vi "PCTrig.vi"(0 "object in":refnum<class "AD2_SDK.lvclass">, 5 "error in (no error)":errorcluster) -> (14 "object out":refnum<class "AD2_SDK.lvclass">, 19 "error out":errorcluster)   [LabVIEW 2019, in "AD2_SDK.lvclass"]
uses:
  AD2_SDK.lvclass
  Olasdwf/Olasdwf.lvlib
panel:
  out "function return":i32
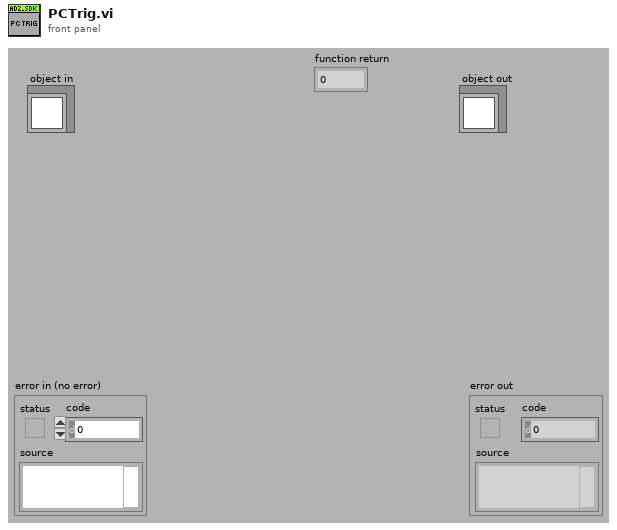
[diagram p1: front panel]
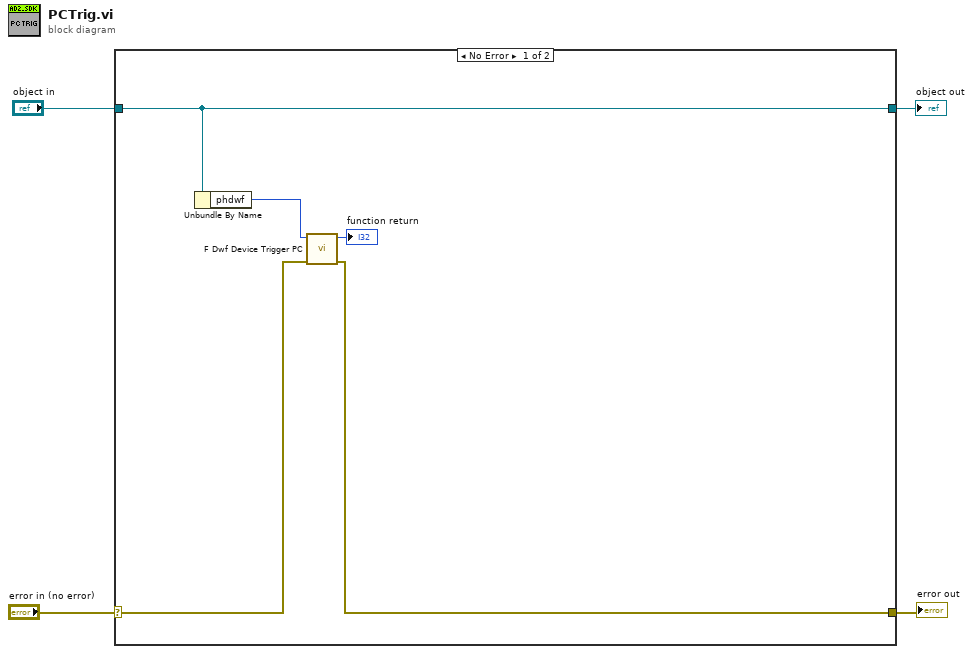
[diagram p0: block diagram]
diagram:
  n1 = case shown="No Error" "error in (no error)" {
    selector: "error in (no error)" -> [w7 w11]
    tunnel: [w6 w11] -> w3
    tunnel: [w9 w10] -> w1
    tunnel: "object in" -> [w9 w10]
    frame No Error {
      n2 = Unbundle By Name(w9) -> ("phdwf"=w8:i32)
      n3 = call "F Dwf Device Trigger PC.vi"("error in (no error)"=w7, "hdwf"=w8) -> ("error out"=w6:errorcluster, "function return"=→"function return":i32)  [unwired: 8 in]
    }
    frame Error {
    }
  }
  "error out" <- w3
  "object out" <- w1
